vi "Update Message Setter.vi"(7 "rpc message name":string, 8 "error in (no error)":errorcluster, 10 "message setter in":refnum<vi>, 11 "rpc messages folder in":refnum<vi>) -> (0 "error out":errorcluster, 2 "message setter out":refnum<vi>, 3 "rpc messages folder out":refnum<vi>)   [LabVIEW 2019, in "gRPC Template Creation Utility.lvlib"]
uses:
  gRPC Template Creation Utility.lvlib
  Oneof API/OneOf Constants/OneOfConstantsEnum.ctl
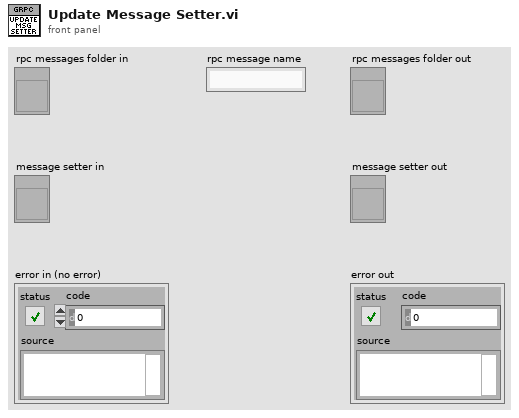
[diagram p1: front panel]
types:
  T1 = typedef "gRPC Template Creation Utility.lvlib/OneOfConstantsEnum.ctl" = enum16{"FlatToRichVIPrefix", "RichToFlatVIPrefix", "FlatTypeDefSuffix"}
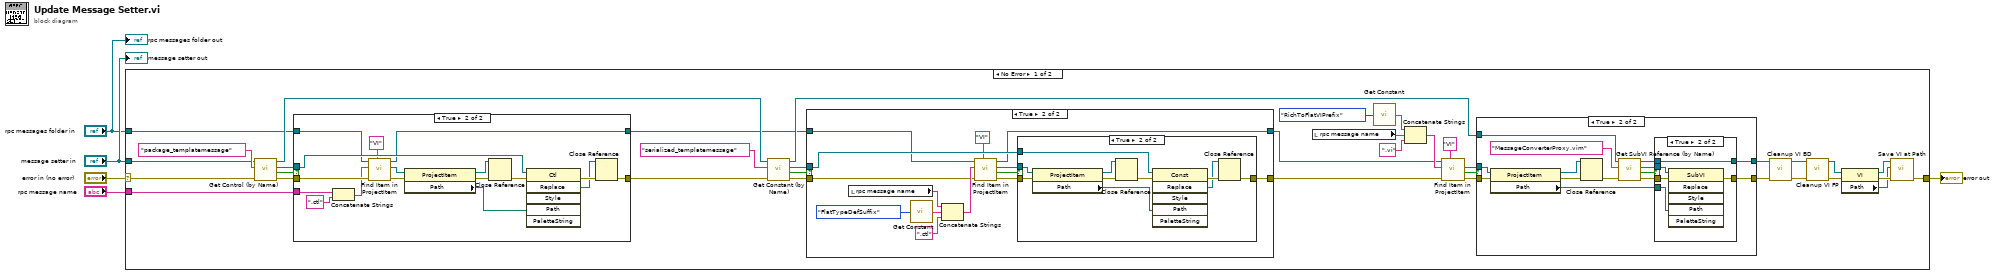
[diagram p0: block diagram]
diagram:
  n1 = case shown="No Error" "error in (no error)" {
    selector: "error in (no error)" -> [w16 w112]
    tunnel: "message setter in" -> [w17 _]
    tunnel: [w13 w112] -> w4
    tunnel: "rpc message name" -> [w12 _]
    tunnel: "rpc messages folder in" -> [w15 _]
    frame No Error {
      n2 = call "Get Control (by Name).vi"("error in (no error)"=w16, "Control Label"="package_templatemessage" ("name/order"), "Owner VI in"=w17) -> ("error out"=w41:errorcluster, "Found ?"=w42:bool, "Control Refnum"=w40:refnum<vi>, "Owner VI out"=w39:refnum<vi>)  [unwired: 5 in]
      n3 = case shown="True" w42 {
        tunnel: [w94 w111] -> w26
        tunnel: w40 -> [_ w108]
        tunnel: w41 -> [w94 w99]
        tunnel: w15 -> [w93 w102]
        tunnel: [w93 w101] -> w14
        tunnel: w12 -> [_ w97]
        frame False {
        }
        frame True {
          n4 = Concatenate Strings(w97, ".ctl" ("string")) -> (w95:string)
          n5 = call "Find Item in ProjectItem.vi"("Item Type"="VI", "error in (no error)"=w99, "Name"=w95, "ProjectItem in"=w102) -> ("error out"=w106:errorcluster, "Item Refnum out"=w107:refnum<vi>, "ProjectItem out"=w101:refnum<vi>)  [unwired: 4 in, 1 out]
          n6 = property class="ProjectItem"(reference=w107, error in=w106) -> (reference out=w105:refnum<vi>, error out=w104:errorcluster, "Path"=w100:path)
          n7 = Close Reference(reference=w105, error in (no error)=w104) -> (error out=w98:errorcluster)
          n8 = invoke class="Ctl" method="Replace"(reference=w108, error in=w98, "Path"=w100) -> (error out=w110:errorcluster, "Replace"=w109:refnum<vi>)  [unwired: 3 in, 4 out]
          n9 = Close Reference(reference=w109, error in (no error)=w110) -> (error out=w111:errorcluster)
        }
      }
      n10 = call "Get Constant (by Name).vi"("error in (no error)"=w26, "Constant Label"="serialized_templatemessage", "Owner VI in"=w39) -> ("error out"=w35:errorcluster, "Found ?"=w36:bool, "Const ref out"=w37:refnum<vi>, "Owner VI out"=w33:refnum<vi>)  [unwired: 5 in]
      n11 = case shown="True" w36 {
        tunnel: [w67 w81] -> w25
        tunnel: w37 -> [_ w80]
        tunnel: w35 -> [w67 w70]
        tunnel: w14 -> [w66 w77]
        tunnel: [w66 w74] -> w24
        frame False {
        }
        frame True {
          n12 = local read "rpc message name"() -> (w79:string)
          n13 = call "Get Constant.vi"("Selection"=OneOfConstantsEnum."FlatTypeDefSuffix") -> ("String"=w68:string)
          n14 = Concatenate Strings(w79, w68, ".ctl" ("string")) -> (w76:string)
          n15 = call "Find Item in ProjectItem.vi"("Item Type"="VI", "error in (no error)"=w70, "Name"=w76, "ProjectItem in"=w77) -> ("error out"=w71:errorcluster, "Found ?"=w72:bool, "Item Refnum out"=w73:refnum<vi>, "ProjectItem out"=w74:refnum<vi>)  [unwired: 4 in]
          n16 = case shown="True" w72 {
            tunnel: [w82 w92] -> w81
            tunnel: w80 -> [_ w89]
            tunnel: w73 -> [_ w88]
            tunnel: w71 -> [w82 w86]
            frame False {
            }
            frame True {
              n17 = property class="ProjectItem"(reference=w88, error in=w86) -> (reference out=w83:refnum<vi>, error out=w85:errorcluster, "Path"=w87:path)
              n18 = Close Reference(reference=w83, error in (no error)=w85) -> (error out=w84:errorcluster)
              n19 = invoke class="Const" method="Replace"(reference=w89, error in=w84, "Path"=w87) -> (error out=w91:errorcluster, "Replace"=w90:refnum<vi>)  [unwired: 3 in, 4 out]
              n20 = Close Reference(reference=w90, error in (no error)=w91) -> (error out=w92:errorcluster)
            }
          }
        }
      }
      n21 = local read "rpc message name"() -> (w32:string)
      n22 = call "Get Constant.vi"("Selection"=OneOfConstantsEnum."RichToFlatVIPrefix") -> ("String"=w21:string)
      n23 = Concatenate Strings(w21, w32, ".vi" ("string")) -> (w30:string)
      n24 = call "Find Item in ProjectItem.vi"("Item Type"="VI", "error in (no error)"=w25, "Name"=w30, "ProjectItem in"=w24) -> ("error out"=w27:errorcluster, "Found ?"=w28:bool, "Item Refnum out"=w23:refnum<vi>)  [unwired: 4 in, 1 out]
      n25 = case shown="True" w28 {
        tunnel: w33 -> [w44 w58]
        tunnel: w27 -> [w43 w51]
        tunnel: [w43 w53] -> w9
        tunnel: [w44 w48] -> w7
        tunnel: w23 -> [_ w52]
        frame False {
        }
        frame True {
          n26 = property class="ProjectItem"(reference=w52, error in=w51) -> (reference out=w45:refnum<vi>, error out=w47:errorcluster, "Path"=w50:path)
          n27 = Close Reference(reference=w45, error in (no error)=w47) -> (error out=w46:errorcluster)
          n28 = call "Get SubVI Reference (by Name).vi"("error in (no error)"=w46, "SubVI Name"="MessageConverterProxy.vim", "Owner VI in"=w58) -> ("error out"=w54:errorcluster, "Found ?"=w56:bool, "SubVI Refnum out"=w55:refnum<vi>, "Owner VI out"=w49:refnum<vi>)  [unwired: 5 in]
          n29 = case shown="True" w56 {
            tunnel: w55 -> [_ w65]
            tunnel: w54 -> [w60 w64]
            tunnel: [w60 w63] -> w53
            tunnel: w50 -> [_ w62]
            tunnel: w49 -> [w59 w61]
            tunnel: [w59 w61] -> w48
            frame False {
            }
            frame True {
              n30 = invoke class="SubVI" method="Replace"(reference=w65, error in=w64, "Path"=w62) -> (error out=w63:errorcluster)  [unwired: 3 in, 5 out]
            }
          }
        }
      }
      n31 = call "Cleanup VI BD.vi"("error in (no error)"=w9, "VI in"=w7) -> ("error out"=w11:errorcluster, "VI out"=w10:refnum<vi>)  [unwired: 8 in]
      n32 = call "Cleanup VI FP.vi"("error in"=w11, "vi in"=w10) -> ("error out"=w8:errorcluster, "vi out"=w6:refnum<vi>)  [unwired: 8 in]
      n33 = property class="VI"(reference=w6, error in=w8) -> (reference out=w20:refnum<vi>, error out=w19:errorcluster, "Path"=w18:path)
      n34 = call "Save VI at Path.vi"("error in (no error)"=w19, "Path"=w18, "VI in"=w20) -> ("error out"=w13:errorcluster)  [unwired: 6 in, 2 out]
    }
    frame Error {
    }
  }
  "error out" <- w4
  "rpc messages folder out" <- "rpc messages folder in"
  "message setter out" <- "message setter in"
